vi "set_z_voltage1.vi"(8 "error in (no error)":errorcluster, 10 "Z Voltage (V)":i16, 11 "PI P123.01 & PiezoDrive TD250 & NI USB 7855R in":refnum<class "PI P123.01 & PiezoDrive TD250 & NI USB 7855R.lvclass">) -> (0 "error out":errorcluster, 3 "PI P123.01 & PiezoDrive TD250 & NI USB 7855R out":refnum<class "PI P123.01 & PiezoDrive TD250 & NI USB 7855R.lvclass">)   [LabVIEW 2020, in "PI P123.01 & PiezoDrive TD250 & NI USB 7855R.lvclass"]
uses:
  PI P123.01 & PiezoDrive TD250 & NI USB 7855R.lvclass
  <vilib>/FPGAPlugInAG/USB-7855R/niLvFpga_Open_USB-7855R.vi
  <vilib>/rvi/interface/common/dynamic/niFpgaDynamicAddResources.vi
  <vilib>/Utility/error.llb/Error Cluster From Error Code.vi
  <vilib>/rvi/errors/niLvFpgaAdjustHostInterfaceError.vi
  <vilib>/rvi/interface/nirviOpenFPGA/nirviOpenFPGA.xnode
  FPGA Bitfiles/afmcontrol_FPGATarget_FPGAmain_od6Q9YeVPLc.lvbitx
  FPGA main.vi
  <vilib>/rvi/interface/nirviReadWriteControl/nirviReadWriteControl.xnode
  NiFpgaLv.dll
  <vilib>/rvi/interface/Simulation/niFpgaSimulationCallBeginRW.vi
panel:
  # "Z voltage is between +/- 10V"
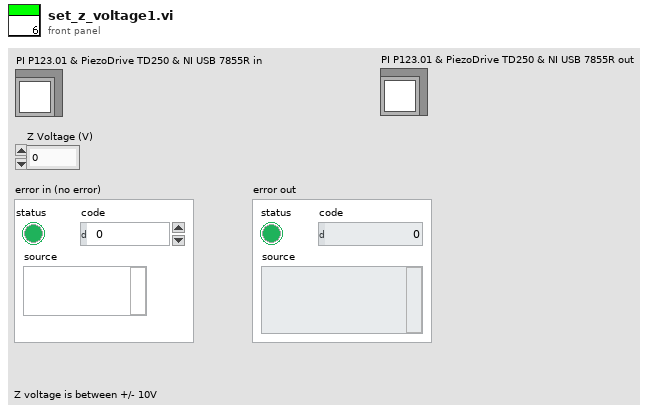
[diagram p1: front panel]
types:
  T1 = enum16{"USB 7855 (AI)", "USB 7855 (AO)", "USB 7855 OEM (AI)", "USB 7855 OEM (AO)", "USB 7856  (AI)", "USB 7856 (AO)", "USB 7856 OEM (AI)", "USB 7856 OEM (AO)"}
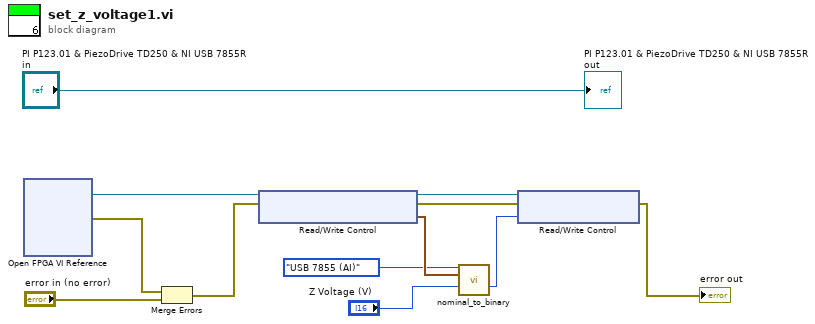
[diagram p0: block diagram]
diagram:
  n1 = xnode "Open FPGA VI Reference"() -> ("FPGA VI Reference Out"=w10:refnum<k20>, "error out"=w11:errorcluster)  [unwired: 2 in]
  n2 = Merge Errors(w11, "error in (no error)") -> (w9:errorcluster)
  n3 = xnode "Read/Write Control"("FPGA VI Reference In"=w10, "error in"=w9) -> ("FPGA VI Reference Out"=w7:refnum<k20>, "error out"=w6:errorcluster, "AO1 Calibration Constants"=w5:cluster{u32, i32})
  n4 = call "nominal_to_binary.vi"("Target Type"=T1."USB 7855 (AI)", "Calibration"=w5, "Nominal Value"="Z Voltage (V)") -> ("Binary Value"=w2:i16)  [unwired: 12 in]
  n5 = xnode "Read/Write Control"("FPGA VI Reference In"=w7, "error in"=w6, "PZT Z Control (Bits)"=w2) -> ("error out"=→"error out":errorcluster)  [unwired: 1 out]
  "PI P123.01 & PiezoDrive TD250 & NI USB 7855R out" <- "PI P123.01 & PiezoDrive TD250 & NI USB 7855R in"
